vi "SetPin.vi"(8 "error in (no error)":errorcluster, 9 "Value":bool, 10 "Led num":u8, 11 "Motorshield in":refnum<class "Motorshield.lvclass">) -> (0 "error out":errorcluster, 3 "Motorshield out":refnum<class "Motorshield.lvclass">)   [LabVIEW 2022 SP3, in "Motorshield.lvlib" / "Motorshield.lvclass"]
uses:
  Motorshield.lvclass
  Motorshield.lvclass/Motorshield.ctl
  pca985/PCA/PCA.lvclass
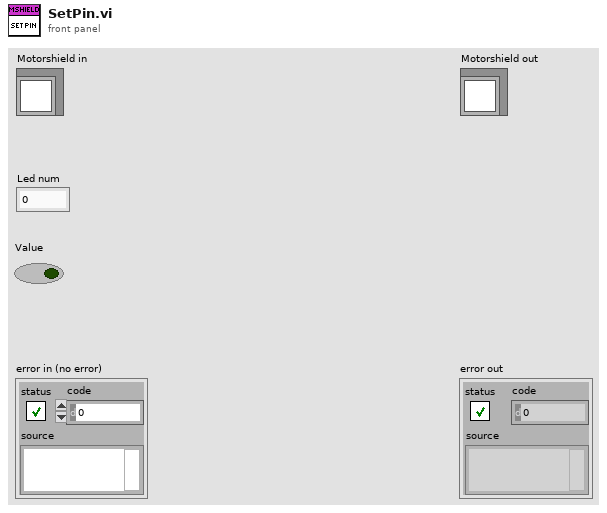
[diagram p1: front panel]
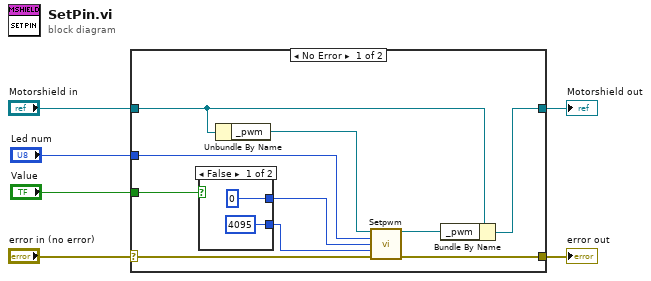
[diagram p0: block diagram]
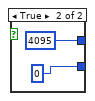
[diagram p2: hidden frame]
diagram:
  n1 = case shown="No Error" "error in (no error)" {
    selector: "error in (no error)" -> [w12 w22]
    tunnel: [w13 w22] -> w5
    tunnel: [w15 w21] -> w3
    tunnel: "Motorshield in" -> [w16 w21]
    tunnel: "Value" -> [w14 _]
    tunnel: "Led num" -> [w9 _]
    frame No Error {
      n2 = case shown="False" w14 {
        tunnel: [0 4095] -> w8
        tunnel: [4095 0] -> w7
        frame False {
        }
        frame True {
        }
      }
      n3 = Unbundle By Name(w16) -> ("_pwm"=w11:refnum<class "PCA.lvclass">)
      n4 = call "Setpwm.vi"("PCA in"=w11, "Led num"=w9, "on"=w8, "off"=w7, "error in (no error)"=w12) -> ("PCA out"=w10:refnum<class "PCA.lvclass">, "error out"=w13:errorcluster)  [unwired: 8 in, 1 out]
      n5 = Bundle By Name(cluster=w16, "_pwm"=w10) -> (w15:refnum<class "Motorshield.lvclass">)
    }
    frame Error {
    }
  }
  "error out" <- w5
  "Motorshield out" <- w3
